vi "Begin.vi"(8 "error in":errorcluster) -> (0 "error out":errorcluster)   [LabVIEW 2014]
doc: "Called before other user functions, this VI is expected to open initial I/O refnums, load in file data, and do all program initialization. Notice that the <B>error out</B> terminal is simply used for data flow. Wiring it to other structures or subVIs ensures that this VI runs first."
uses:
  <vilib>/Rock Robotics/WPI/DriverStation/WPI_DriverStationRobotMode2.ctl
  <vilib>/Rock Robotics/SystemInterfaces/DIO/FPGA_DIOChannel.ctl
  <vilib>/Rock Robotics/WPI/Encoder/WPI_EncoderType.ctl
  <vilib>/Rock Robotics/SystemInterfaces/DIO/FPGA_DIOPWMChannel.ctl
  <vilib>/Rock Robotics/WPI/Joystick/WPI_JoystickDeviceEnum.ctl
  <vilib>/Rock Robotics/WPI/Solenoid/WPI_SolenoidChannel.ctl
  Robot Global Data.vi
  <vilib>/Rock Robotics/Network Tables/SD Write String Array.vi
  <vilib>/Rock Robotics/WPI/Counter/WPI_CounterDigitalInputToDigitalSource.vi
  <vilib>/Rock Robotics/WPI/RobotDrive/WPI_RobotDriveOpen4MotorWithTalonSRX.vi
  <vilib>/Rock Robotics/WPI/Solenoid/WPI_SolenoidOpenDouble.vi
  <vilib>/Rock Robotics/WPI/MotorControl/WPI_MotorControlOpen TalonSRX.vi
  <vilib>/Rock Robotics/WPI/Compressor/WPI_CompressorGetSetRefNum.vi
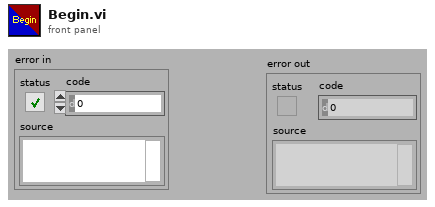
[diagram p1: front panel]
types:
  T1 = typedef "WPI_EncoderType.ctl" = enum16{"1x", "2x", "4x"}
  T2 = typedef "FPGA_DIOChannel.ctl" = enum8{"DIO 0", "DIO 1", "DIO 2", "DIO 3", "DIO 4", "DIO 5", "DIO 6", "DIO 7", "DIO 8", "DIO 9", "DIO MXP 0", "DIO MXP 1", "DIO MXP 2", "DIO MXP 3", "DIO MXP 4", "DIO MXP 5", "DIO MXP 6", "DIO MXP 7", "DIO MXP 8", "DIO MXP 9", "DIO MXP 10", "DIO MXP 11", "DIO MXP 12", "DIO MXP 13", "DIO MXP 14", "DIO MXP 15", "Invalid"}
  T3 = typedef "FPGA_DIOPWMChannel.ctl" = enum8{"PWM 0", "PWM 1", "PWM 2", "PWM 3", "PWM 4", "PWM 5", "PWM 6", "PWM 7", "PWM 8", "PWM 9", "PWM MXP 0", "PWM MXP 1", "PWM MXP 2", "PWM MXP 3", "PWM MXP 4", "PWM MXP 5", "PWM MXP 6", "PWM MXP 7", "PWM MXP 8", "PWM MXP 9", "Invalid"}
  T4 = typedef "WPI_SolenoidChannel.ctl" = enum8{"Solenoid 0", "Solenoid 1", "Solenoid 2", "Solenoid 3", "Solenoid 4", "Solenoid 5", "Solenoid 6", "Solenoid 7", "Invalid"}
  T5 = typedef "WPI_JoystickDeviceEnum.ctl" = enum16{"USB 0", "USB 1", "USB 2", "USB 3", "USB 4", "USB 5"}
  T6 = typedef "WPI_DriverStationRobotMode2.ctl" = enum16{"Autonomous Disabled", "Autonomous Enabled", "Teleop Disabled", "Teleop Enabled", "Disconnected", "Finish", "Test Disabled", "Test Enabled", "Emergency Stopped"}
  T7 = typedef "WPI_DigitalInputDevRef.ctl" = cluster{"DevStatus":errorcluster, "DIO Channel":T2, "Controller":T8}
  T8 = typedef "FPGA_TypedefDigitalModule.ctl" = enum16{"Controller 1"}
  T9 = typedef "WPI_JoystickDevRef.ctl" = cluster{"Device":T5}
  T10 = typedef "WPI_CompressorDevRef.ctl" = cluster{"DevStatus":errorcluster, "Pneumatics Control Module":u8}
  T11 = typedef "WPI_SolenoidDevRef.ctl" = cluster{"DevStatus":errorcluster, "Pneumatics Control Module":u8, "Forward Solenoid Channel":T4, "Reverse Solenoid Channel":T4}
  T12 = typedef "WPI_MotorControlDeviceRef.ctl" = cluster{"DeviceStatus":errorcluster, "Type":T13, "PWM":cluster{"Controller":T8, "PWM Channel":T3, "DeadBand":T14}, "CAN":cluster{"Device Number":u8, "Control Mode":T15, "Semaphore":T16, "Max Vout":dbl, "TalonSRX Control Mode":T17}, "Invert":bool, "TransformRef":T18, "InvTransformRef":T18}
  T13 = typedef "WPI_MotorControlType.ctl" = enum16{"PWM", "CAN", "CANTalonSRX"}
  T14 = typedef "WPI_PWMDeadband.ctl" = cluster{"Name":string, "maxPositivePwm":i32, "minPositivePwm":i32, "centerPwm":i32, "maxNegativePwm":i32, "minNegativePwm":i32, "angularRange":u16}
  T15 = typedef "WPI_CANJaguar_ControlMode.ctl" = enum8{"Percent VBus", "Current", "Speed", "Position", "Voltage"}
  T16 = typedef "Semaphore RefNum" = refnum<k1>
  T17 = typedef "WPI_CANTalonSRX_APIControlMode.ctl" = enum8{"Percent VBus", "Speed", "Position", "Slave", "Unchanged / Invalid"}
  T18 = typedef "WPI_PWMTransform_ConPane.ctl" = refnum<vi>
  T19 = typedef "FPGA_CounterEncoderSourceConvertionLVSourceType.ctl" = cluster{"DevStatus":errorcluster, "AnalogTriggerMode?":bool, "DigitalMode":cluster{"Controller":T8, "DIO Channel":T20}, "AnalogTriggerMode":cluster{"AnalogTriggerIndex":T21, "OutputType":T22}}
  T20 = typedef "FPGA_DIODigitalSourceChannel.ctl" = enum8{"DIO 0", "DIO 1", "DIO 2", "DIO 3", "DIO 4", "DIO 5", "DIO 6", "DIO 7", "DIO 8", "DIO 9", "DIO MXP 0", "DIO MXP 1", "DIO MXP 2", "DIO MXP 3", "DIO MXP 4", "DIO MXP 5", "DIO MXP 6", "DIO MXP 7", "DIO MXP 8", "DIO MXP 9", "DIO MXP 10", "DIO MXP 11", "DIO MXP 12", "DIO MXP 13", "DIO MXP 14", "DIO MXP 15", "Disabled"}
  T21 = typedef "FPGA_AnalogTriggerIndex.ctl" = enum8{"Trig 0", "Trig 1", "Trig 2", "Trig 3", "Trig 4", "Trig 5", "Trig 6", "Trig 7", "Invalid"}
  T22 = typedef "FPGA_AnalogTriggerOutType.ctl" = enum16{"InWindow", "TriggerState", "Rising", "Falling"}
  T23 = typedef "WPI_RobotDriveDevRef.ctl" = cluster{"DevStatus":errorcluster, "Motors[]":T12[], "Square Inputs":bool, "Max Output":dbl}
  T24 = typedef "WPI_EncoderDevRef.ctl" = cluster{"DevStatus":errorcluster, "EncoderIndex":T25, "CounterIndex":T26, "DistancePerCount":dbl, "Decoding Type":T1}
  T25 = typedef "FPGA_EncoderIdx.ctl" = enum8{"Enc 0", "Enc 1", "Enc 2", "Enc 3", "Enc 4", "Enc 5", "Enc 6", "Enc 7", "Invalid"}
  T26 = typedef "FPGA_CounterCtrSystemIndex.ctl" = enum8{"Ctr 0", "Ctr 1", "Ctr 2", "Ctr 3", "Ctr 4", "Ctr 5", "Ctr 6", "Ctr 7", "Invalid"}
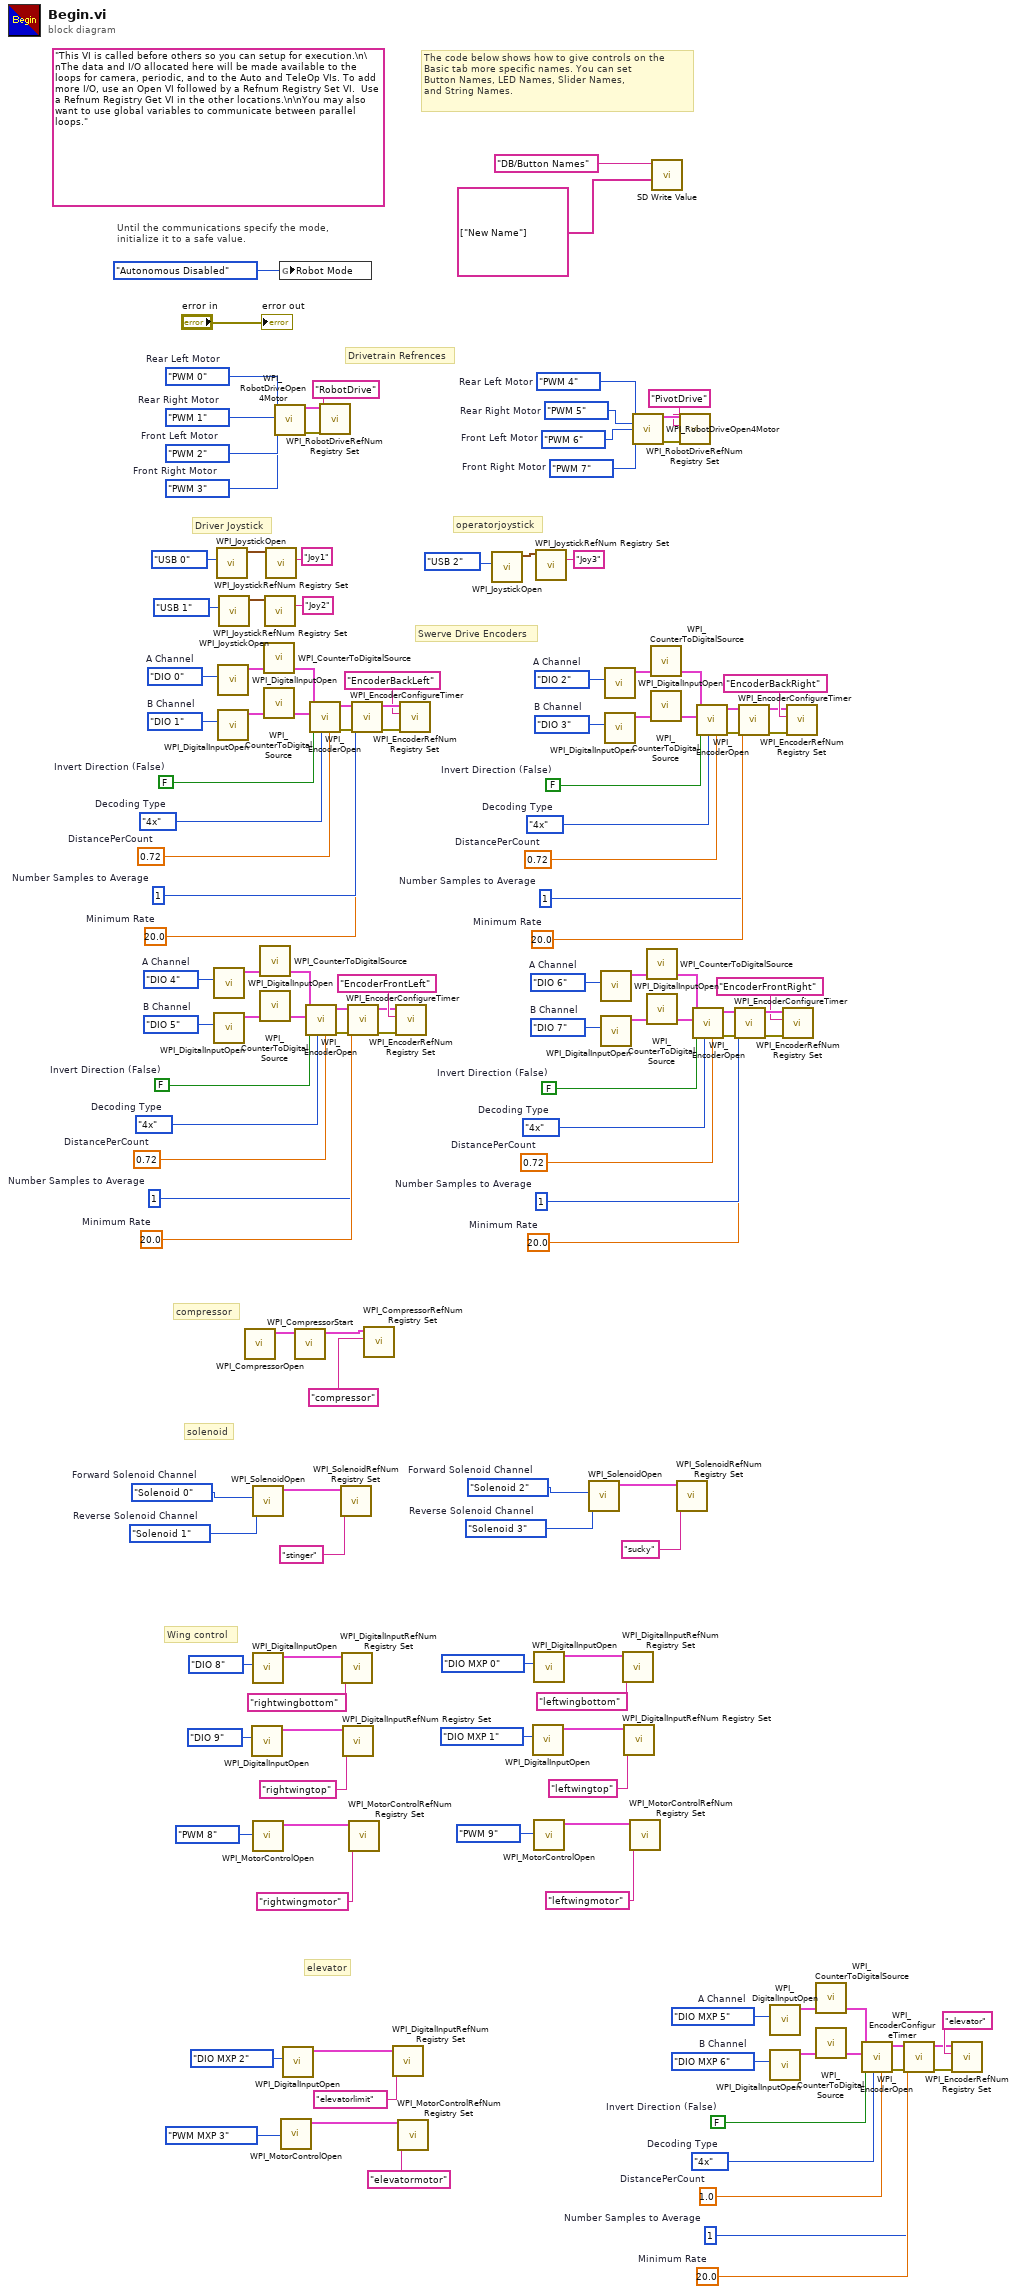
[diagram p0: block diagram]
diagram:
  w13 = 20.0  # Minimum Rate
  w12 = u8 1  # Number Samples to Average
  w9 = 1.0  # DistancePerCount
  w7 = FALSE  # Invert Direction (False)
  w8 = WPI_EncoderType."4x"  # Decoding Type
  w1 = FPGA_DIOChannel."DIO MXP 6"  # B Channel
  w2 = FPGA_DIOChannel."DIO MXP 5"  # A Channel
  w44 = WPI_SolenoidChannel."Solenoid 3"  # Reverse Solenoid Channel
  w43 = WPI_SolenoidChannel."Solenoid 2"  # Forward Solenoid Channel
  w48 = WPI_SolenoidChannel."Solenoid 1"  # Reverse Solenoid Channel
  w49 = WPI_SolenoidChannel."Solenoid 0"  # Forward Solenoid Channel
  w62 = FPGA_DIOPWMChannel."PWM 7"  # Front Right Motor
  w63 = FPGA_DIOPWMChannel."PWM 6"  # Front Left Motor
  w64 = FPGA_DIOPWMChannel."PWM 5"  # Rear Right Motor
  w65 = FPGA_DIOPWMChannel."PWM 4"  # Rear Left Motor
  w71 = FPGA_DIOPWMChannel."PWM 3"  # Front Right Motor
  w72 = FPGA_DIOPWMChannel."PWM 2"  # Front Left Motor
  w73 = FPGA_DIOPWMChannel."PWM 1"  # Rear Right Motor
  w74 = FPGA_DIOPWMChannel."PWM 0"  # Rear Left Motor
  w94 = 20.0  # Minimum Rate
  w95 = u8 1  # Number Samples to Average
  w98 = 0.72  # DistancePerCount
  w100 = FALSE  # Invert Direction (False)
  w99 = WPI_EncoderType."4x"  # Decoding Type
  w106 = FPGA_DIOChannel."DIO 7"  # B Channel
  w105 = FPGA_DIOChannel."DIO 6"  # A Channel
  w87 = 20.0  # Minimum Rate
  w86 = u8 1  # Number Samples to Average
  w83 = 0.72  # DistancePerCount
  w81 = FALSE  # Invert Direction (False)
  w82 = WPI_EncoderType."4x"  # Decoding Type
  w75 = FPGA_DIOChannel."DIO 5"  # B Channel
  w76 = FPGA_DIOChannel."DIO 4"  # A Channel
  w119 = 20.0  # Minimum Rate
  w118 = u8 1  # Number Samples to Average
  w115 = 0.72  # DistancePerCount
  w113 = FALSE  # Invert Direction (False)
  w114 = WPI_EncoderType."4x"  # Decoding Type
  w107 = FPGA_DIOChannel."DIO 3"  # B Channel
  w108 = FPGA_DIOChannel."DIO 2"  # A Channel
  w126 = 20.0  # Minimum Rate
  w127 = u8 1  # Number Samples to Average
  w130 = 0.72  # DistancePerCount
  w132 = FALSE  # Invert Direction (False)
  w131 = WPI_EncoderType."4x"  # Decoding Type
  w138 = FPGA_DIOChannel."DIO 1"  # B Channel
  w137 = FPGA_DIOChannel."DIO 0"  # A Channel
  (unwired) "This VI is called before others so you can setup for execution.\n\nThe data and I/O allocated here will be made available to the loops for camera, periodic, and to the Auto and TeleOp VIs. To add more I/O, use an Open VI followed by a Refnum Registry Set VI.  Use a Refnum Registry Get VI in the other locations.\n\nYou may also want to use global variables to communicate between parallel loops."
  # "elevator"
  # "Wing control"
  # "operatorjoystick"
  # "solenoid"
  # "compressor"
  # "Driver Joystick"
  # "Drivetrain Refrences"
  # "Swerve Drive Encoders"
  # "The code below shows how to give controls on the\nBasic tab more specific names. You can set\nButton Names, LED Names, Slider Names,\nand String Names."
  # "Until the communications specify the mode,\ninitialize it to a safe value."
  n1 = call <vilib>:"WPI_DigitalInputOpen.vi"("DIO Channel"=w76) -> ("DigitalInputDevRef"=w79:T7)  [unwired: 2 in, 8 out]
  n2 = call <vilib>:"WPI_DigitalInputOpen.vi"("DIO Channel"=w75) -> ("DigitalInputDevRef"=w78:T7)  [unwired: 2 in, 8 out]
  n3 = call <vilib>:"WPI_JoystickOpen.vi"("JoystickDevice"=WPI_JoystickDeviceEnum."USB 0") -> ("JoystickDevRef"=w57:T9)  [unwired: 10 in]
  n4 = call <vilib>:"WPI_DigitalInputOpen.vi"("DIO Channel"=w137) -> ("DigitalInputDevRef"=w134:T7)  [unwired: 2 in, 8 out]
  n5 = call <vilib>:"WPI_DigitalInputOpen.vi"("DIO Channel"=w138) -> ("DigitalInputDevRef"=w135:T7)  [unwired: 2 in, 8 out]
  n6 = call <vilib>:"WPI_JoystickOpen.vi"("JoystickDevice"=WPI_JoystickDeviceEnum."USB 1") -> ("JoystickDevRef"=w58:T9)  [unwired: 10 in]
  n7 = call <vilib>:"WPI_CompressorOpen.vi"() -> ("CompressorDevRef"=w54:T10)  [unwired: 14 in, 1 out]
  n8 = call <vilib>:"WPI_DigitalInputOpen.vi"("DIO Channel"=FPGA_DIOChannel."DIO 9") -> ("DigitalInputDevRef"=w39:T7)  [unwired: 9 in, 1 out]
  n9 = call-poly <vilib>:"WPI_SolenoidOpen.vi"("Reverse Solenoid Channel"=w48, "Forward Solenoid Channel"=w49) -> ("SolenoidDevRef"=w51:T11)  [unwired: 2 in, 7 out]
  n10 = call <vilib>:"WPI_DigitalInputOpen.vi"("DIO Channel"=FPGA_DIOChannel."DIO 8") -> ("DigitalInputDevRef"=w40:T7)  [unwired: 9 in, 1 out]
  n11 = call-poly <vilib>:"WPI_MotorControlOpen.vi"("PWM Channel"=FPGA_DIOPWMChannel."PWM 8") -> ("MotorControlDeviceRef"=w34:T12)  [unwired: 9 in, 1 out]
  n12 = call-poly <vilib>:"WPI_CounterToDigitalSource.vi"("DigitalInputDevRef"=w79) -> ("Digital Source"=w80:T19)  [unwired: 6 out]
  n13 = call-poly <vilib>:"WPI_CounterToDigitalSource.vi"("DigitalInputDevRef"=w78) -> ("Digital Source"=w77:T19)  [unwired: 6 out]
  n14 = call-poly <vilib>:"WPI_CounterToDigitalSource.vi"("DigitalInputDevRef"=w134) -> ("Digital Source"=w133:T19)  [unwired: 6 out]
  n15 = call-poly <vilib>:"WPI_CounterToDigitalSource.vi"("DigitalInputDevRef"=w135) -> ("Digital Source"=w136:T19)  [unwired: 6 out]
  n16 = call <vilib>:"WPI_JoystickRefNum Registry Set.vi"("refnum name"="Joy2", "JoystickDevRef"=w58) -> ()  [unwired: 8 in, 2 out]
  n17 = call <vilib>:"WPI_JoystickRefNum Registry Set.vi"("refnum name"="Joy1", "JoystickDevRef"=w57) -> ()  [unwired: 8 in, 2 out]
  n18 = call-poly <vilib>:"WPI_RobotDriveOpen4Motor.vi"("Rear Left Motor"=w74, "Rear Right Motor"=w73, "Front Left Motor"=w72, "Front Right Motor"=w71) -> ("RobotDriveDevRef"=w69:T23, "error out"=w70:errorcluster)  [unwired: 10 in]
  n19 = global write "Robot Global Data.vi" "Robot Mode"(WPI_DriverStationRobotMode2."Autonomous Disabled" ("Robot Mode")) -> ()
  n20 = call-poly <vilib>:"WPI_MotorControlOpen.vi"("PWM Channel"=FPGA_DIOPWMChannel."PWM MXP 3") -> ("MotorControlDeviceRef"=w20:T12)  [unwired: 9 in, 1 out]
  n21 = call <vilib>:"WPI_DigitalInputOpen.vi"("DIO Channel"=FPGA_DIOChannel."DIO MXP 2") -> ("DigitalInputDevRef"=w22:T7)  [unwired: 9 in, 1 out]
  n22 = call <vilib>:"WPI_CompressorStart.vi"("CompressorDevRef"=w54) -> ("CompressorDevRef"=w53:T10)  [unwired: 1 in, 9 out]
  n23 = call <vilib>:"WPI_EncoderOpen.vi"("DistancePerCount"=w83, "Decoding Type"=w82, "Invert Direction (False)"=w81, "BSource"=w77, "ASource"=w80) -> ("error out"=w84:errorcluster, "EncoderDevRef"=w85:T24)  [unwired: 3 in, 2 out]
  n24 = call <vilib>:"WPI_EncoderOpen.vi"("DistancePerCount"=w130, "Decoding Type"=w131, "Invert Direction (False)"=w132, "BSource"=w136, "ASource"=w133) -> ("error out"=w129:errorcluster, "EncoderDevRef"=w128:T24)  [unwired: 3 in, 2 out]
  n25 = call <vilib>:"WPI_RobotDriveRefNum Registry Set.vi"("error in (no error)"=w70, "refnum name"="RobotDrive", "RobotDriveDevRef"=w69) -> ()  [unwired: 7 in, 2 out]
  n26 = call <vilib>:"WPI_SolenoidRefNum Registry Set.vi"("refnum name"="stinger", "SolenoidDevRef"=w51) -> ()  [unwired: 8 in, 2 out]
  n27 = call <vilib>:"WPI_DigitalInputRefNum Registry Set.vi"("refnum name"="rightwingbottom", "DigitalInputDevRef"=w40) -> ()  [unwired: 8 in, 2 out]
  n28 = call <vilib>:"WPI_DigitalInputRefNum Registry Set.vi"("refnum name"="rightwingtop", "DigitalInputDevRef"=w39) -> ()  [unwired: 8 in, 2 out]
  n29 = call <vilib>:"WPI_EncoderConfigureTimer.vi"("error in (no error)"=w84, "Number Samples to Average"=w86, "Minimum Rate"=w87, "EncoderDevRef"=w85) -> ("error out"=w88:errorcluster, "EncoderDevRef"=w89:T24)  [unwired: 6 in]
  n30 = call <vilib>:"WPI_MotorControlRefNum Registry Set.vi"("refnum name"="rightwingmotor", "MotorControlDevRef"=w34) -> ()  [unwired: 8 in, 2 out]
  n31 = call <vilib>:"WPI_EncoderConfigureTimer.vi"("error in (no error)"=w129, "Number Samples to Average"=w127, "Minimum Rate"=w126, "EncoderDevRef"=w128) -> ("error out"=w125:errorcluster, "EncoderDevRef"=w124:T24)  [unwired: 6 in]
  n32 = call <vilib>:"WPI_CompressorRefNum Registry Set.vi"("refnum name"="compressor", "CompressorDevRef"=w53) -> ()  [unwired: 8 in, 2 out]
  n33 = call <vilib>:"WPI_DigitalInputRefNum Registry Set.vi"("refnum name"="elevatorlimit", "DigitalInputDevRef"=w22) -> ()  [unwired: 8 in, 2 out]
  n34 = call <vilib>:"WPI_EncoderRefNum Registry Set.vi"("error in (no error)"=w88, "refnum name"="EncoderFrontLeft", "EncoderDevRef"=w89) -> ()  [unwired: 7 in, 2 out]
  n35 = call <vilib>:"WPI_MotorControlRefNum Registry Set.vi"("refnum name"="elevatormotor", "MotorControlDevRef"=w20) -> ()  [unwired: 8 in, 2 out]
  n36 = call <vilib>:"WPI_EncoderRefNum Registry Set.vi"("error in (no error)"=w125, "refnum name"="EncoderBackLeft", "EncoderDevRef"=w124) -> ()  [unwired: 7 in, 2 out]
  n37 = call <vilib>:"WPI_JoystickOpen.vi"("JoystickDevice"=WPI_JoystickDeviceEnum."USB 2") -> ("JoystickDevRef"=w46:T9)  [unwired: 10 in]
  n38 = call <vilib>:"WPI_DigitalInputOpen.vi"("DIO Channel"=FPGA_DIOChannel."DIO MXP 1") -> ("DigitalInputDevRef"=w24:T7)  [unwired: 9 in, 1 out]
  n39 = call <vilib>:"WPI_DigitalInputOpen.vi"("DIO Channel"=FPGA_DIOChannel."DIO MXP 0") -> ("DigitalInputDevRef"=w23:T7)  [unwired: 9 in, 1 out]
  n40 = call-poly <vilib>:"WPI_MotorControlOpen.vi"("PWM Channel"=FPGA_DIOPWMChannel."PWM 9") -> ("MotorControlDeviceRef"=w29:T12)  [unwired: 9 in, 1 out]
  n41 = call <vilib>:"WPI_JoystickRefNum Registry Set.vi"("refnum name"="Joy3", "JoystickDevRef"=w46) -> ()  [unwired: 8 in, 2 out]
  n42 = call-poly <vilib>:"WPI_SolenoidOpen.vi"("Reverse Solenoid Channel"=w44, "Forward Solenoid Channel"=w43) -> ("SolenoidDevRef"=w41:T11)  [unwired: 2 in, 7 out]
  n43 = call <vilib>:"WPI_DigitalInputOpen.vi"("DIO Channel"=w105) -> ("DigitalInputDevRef"=w102:T7)  [unwired: 2 in, 8 out]
  n44 = call <vilib>:"WPI_DigitalInputOpen.vi"("DIO Channel"=w106) -> ("DigitalInputDevRef"=w103:T7)  [unwired: 2 in, 8 out]
  n45 = call <vilib>:"WPI_DigitalInputOpen.vi"("DIO Channel"=w108) -> ("DigitalInputDevRef"=w111:T7)  [unwired: 2 in, 8 out]
  n46 = call <vilib>:"WPI_DigitalInputOpen.vi"("DIO Channel"=w107) -> ("DigitalInputDevRef"=w110:T7)  [unwired: 2 in, 8 out]
  n47 = call <vilib>:"WPI_DigitalInputRefNum Registry Set.vi"("refnum name"="leftwingbottom", "DigitalInputDevRef"=w23) -> ()  [unwired: 8 in, 2 out]
  n48 = call <vilib>:"WPI_DigitalInputRefNum Registry Set.vi"("refnum name"="leftwingtop", "DigitalInputDevRef"=w24) -> ()  [unwired: 8 in, 2 out]
  n49 = call <vilib>:"WPI_MotorControlRefNum Registry Set.vi"("refnum name"="leftwingmotor", "MotorControlDevRef"=w29) -> ()  [unwired: 8 in, 2 out]
  n50 = call-poly <vilib>:"WPI_RobotDriveOpen4Motor.vi"("Rear Left Motor"=w65, "Rear Right Motor"=w64, "Front Left Motor"=w63, "Front Right Motor"=w62) -> ("RobotDriveDevRef"=w66:T23, "error out"=w67:errorcluster)  [unwired: 10 in]
  n51 = call-poly <vilib>:"WPI_CounterToDigitalSource.vi"("DigitalInputDevRef"=w102) -> ("Digital Source"=w101:T19)  [unwired: 6 out]
  n52 = call-poly <vilib>:"WPI_CounterToDigitalSource.vi"("DigitalInputDevRef"=w103) -> ("Digital Source"=w104:T19)  [unwired: 6 out]
  n53 = call-poly <vilib>:"WPI_CounterToDigitalSource.vi"("DigitalInputDevRef"=w111) -> ("Digital Source"=w112:T19)  [unwired: 6 out]
  n54 = call-poly <vilib>:"WPI_CounterToDigitalSource.vi"("DigitalInputDevRef"=w110) -> ("Digital Source"=w109:T19)  [unwired: 6 out]
  n55 = call-poly <vilib>:"SD Write Value.vi"("String Array"=string[] ["New Name"], "Name"="DB/Button Names") -> ()  [unwired: 8 in, 2 out]
  n56 = call <vilib>:"WPI_SolenoidRefNum Registry Set.vi"("refnum name"="sucky", "SolenoidDevRef"=w41) -> ()  [unwired: 8 in, 2 out]
  n57 = call <vilib>:"WPI_RobotDriveRefNum Registry Set.vi"("error in (no error)"=w67, "refnum name"="PivotDrive", "RobotDriveDevRef"=w66) -> ()  [unwired: 7 in, 2 out]
  n58 = call <vilib>:"WPI_EncoderOpen.vi"("DistancePerCount"=w98, "Decoding Type"=w99, "Invert Direction (False)"=w100, "BSource"=w104, "ASource"=w101) -> ("error out"=w97:errorcluster, "EncoderDevRef"=w96:T24)  [unwired: 3 in, 2 out]
  n59 = call <vilib>:"WPI_EncoderOpen.vi"("DistancePerCount"=w115, "Decoding Type"=w114, "Invert Direction (False)"=w113, "BSource"=w109, "ASource"=w112) -> ("error out"=w116:errorcluster, "EncoderDevRef"=w117:T24)  [unwired: 3 in, 2 out]
  n60 = call <vilib>:"WPI_EncoderConfigureTimer.vi"("error in (no error)"=w97, "Number Samples to Average"=w95, "Minimum Rate"=w94, "EncoderDevRef"=w96) -> ("error out"=w93:errorcluster, "EncoderDevRef"=w92:T24)  [unwired: 6 in]
  n61 = call <vilib>:"WPI_EncoderConfigureTimer.vi"("error in (no error)"=w116, "Number Samples to Average"=w118, "Minimum Rate"=w119, "EncoderDevRef"=w117) -> ("error out"=w120:errorcluster, "EncoderDevRef"=w121:T24)  [unwired: 6 in]
  n62 = call <vilib>:"WPI_DigitalInputOpen.vi"("DIO Channel"=w2) -> ("DigitalInputDevRef"=w5:T7)  [unwired: 2 in, 8 out]
  n63 = call <vilib>:"WPI_DigitalInputOpen.vi"("DIO Channel"=w1) -> ("DigitalInputDevRef"=w4:T7)  [unwired: 2 in, 8 out]
  n64 = call <vilib>:"WPI_EncoderRefNum Registry Set.vi"("error in (no error)"=w93, "refnum name"="EncoderFrontRight", "EncoderDevRef"=w92) -> ()  [unwired: 7 in, 2 out]
  n65 = call <vilib>:"WPI_EncoderRefNum Registry Set.vi"("error in (no error)"=w120, "refnum name"="EncoderBackRight", "EncoderDevRef"=w121) -> ()  [unwired: 7 in, 2 out]
  n66 = call-poly <vilib>:"WPI_CounterToDigitalSource.vi"("DigitalInputDevRef"=w5) -> ("Digital Source"=w6:T19)  [unwired: 6 out]
  n67 = call-poly <vilib>:"WPI_CounterToDigitalSource.vi"("DigitalInputDevRef"=w4) -> ("Digital Source"=w3:T19)  [unwired: 6 out]
  n68 = call <vilib>:"WPI_EncoderOpen.vi"("DistancePerCount"=w9, "Decoding Type"=w8, "Invert Direction (False)"=w7, "BSource"=w3, "ASource"=w6) -> ("error out"=w10:errorcluster, "EncoderDevRef"=w11:T24)  [unwired: 3 in, 2 out]
  n69 = call <vilib>:"WPI_EncoderConfigureTimer.vi"("error in (no error)"=w10, "Number Samples to Average"=w12, "Minimum Rate"=w13, "EncoderDevRef"=w11) -> ("error out"=w14:errorcluster, "EncoderDevRef"=w15:T24)  [unwired: 6 in]
  n70 = call <vilib>:"WPI_EncoderRefNum Registry Set.vi"("error in (no error)"=w14, "refnum name"="elevator", "EncoderDevRef"=w15) -> ()  [unwired: 7 in, 2 out]
  "error out" <- "error in"
